vi "Sensor Group 6 to Sensor Group 6 (graphical).vi"(3 "Net Angle (deg)":i32, 4 "Net Dist (mm)":i32, 6 "iRobot Sensor Group 6":T1={"Bumps + Wheel Drops"={"Wheeldrop Caster"=FALSE, "Wheeldrop Left"=FALSE, "Wheeldrop Right"=FALSE, "Bump Left"=FALSE, "Bump Right"=FALSE}, "Wall"=FALSE, "Cliff Left"=FALSE, "Cliff Front Left"=FALSE, "Cliff Front Right"=FALSE, "Cliff Right"=FALSE, "Wall Signal"=0, "Cliff Left Signal"=0, "Cliff Front Left Signal"=0, "Cliff Front Right Signal"=0, "Cliff Right Signal"=0, "Buttons"={"Advance"=FALSE, "Play"=FALSE}, "Virtual Wall"=FALSE, "# Stream Packets"=0, "Requested Velocity (mm/s)"=0, "Requested Radius (mm)"=0, "Requested Right Wheel Velocity (mm/s)"=0, "Requested Left Wheel Velocity (mm/s)"=0, "Distance (mm)"=0, "Angle (deg)"=0, "Song Playing"=FALSE, "Song Number"=0, "Charging State"=enum."Not Charging", "Voltage (mV)"=0, "Current (mA)"=0, "Battery Temperature (deg C)"=0, "Battery Charge (mAh)"=0, "Battery Capacity (mAh)"=0, "Charging Sources"={"Internal Charger"=FALSE, "Home Base"=FALSE}, "OI Mode"=enum."Off", "Digital Inputs"={"Digital Input 0"=FALSE, "Digital Input 1"=FALSE, "Digital Input 2"=FALSE, "Digital Input 3"=FALSE, "Device Detect"=FALSE}, "Drivers & Wheel Overcurrent"={"Low-Side Driver 0"=FALSE, "Low-Side Driver 1"=FALSE, "Low-Side Driver 2"=FALSE, "Left Wheel"=FALSE, "Right Wheel"=FALSE}, "Analog Signal"=0, "Infrared"=255} {"Infrared" format="%02x"}) -> (1 "iRobot Sensors (graphical)":T9={"Caster Wheel Drop"=FALSE, "Left Wheel Drop"=FALSE, "Right Wheel Drop"=FALSE, "Left Bump"=FALSE, "Right Bump"=FALSE, "Left Cliff"=FALSE, "Front Left Cliff"=FALSE, "Front Right Cliff"=FALSE, "Right Cliff"=FALSE, "Wall"=FALSE, "Left Wheel Overcurrent"=FALSE, "Right Wheel Overcurrent"=FALSE, "Infrared"=255, "Play"=FALSE, "Advance"=FALSE, "Net Dist (mm)"=0, "Net Angle (deg)"=0, "Charging State"=enum."Not Charging", "Voltage (mV)"=0, "Current (mA)"=0, "Battery Temperature (C)"=0, "Battery Charge (mAh)"=0, "Battery Capacity (mAh)"=255, "Wall (mm)"=0, "Left Cliff"=0, "Front Left Cliff"=0, "Front Right Cliff"=0, "Right Cliff"=0, "OI Mode"=enum."Off", "Song Number"=0, "Song Playing"=FALSE, "Power"=FALSE, "Left Wheel (mm/s)"=0, "Right Wheel (mm/s)"=0} {"Infrared" format="%02x"; "Right Wheel (mm/s)" scale=-500.0..500.0; "Left Wheel (mm/s)" scale=-500.0..500.0})   [LabVIEW 2014]
uses:
  Sensor Group 6 (graphical).ctl
  Charging State.ctl
  OI Mode.ctl
  Sensor Group 6.ctl
  Bumps + Wheel Drops.ctl
  Buttons.ctl
  Charging Sources Available.ctl
  Cargo Bay Digital Inputs.ctl
  Low-Side Driver + Wheel Overcurrent.ctl
panel:
  # "Electrical: charging, battery, OI mode"
  # "Sensors: bump, cliff, button, wheel drop, wall, virtual wall"
  # "Motion: distance, angle, requested velocity"
  # "Cargo Bay: I/O, overcurrent, infrared"
  # "Song"
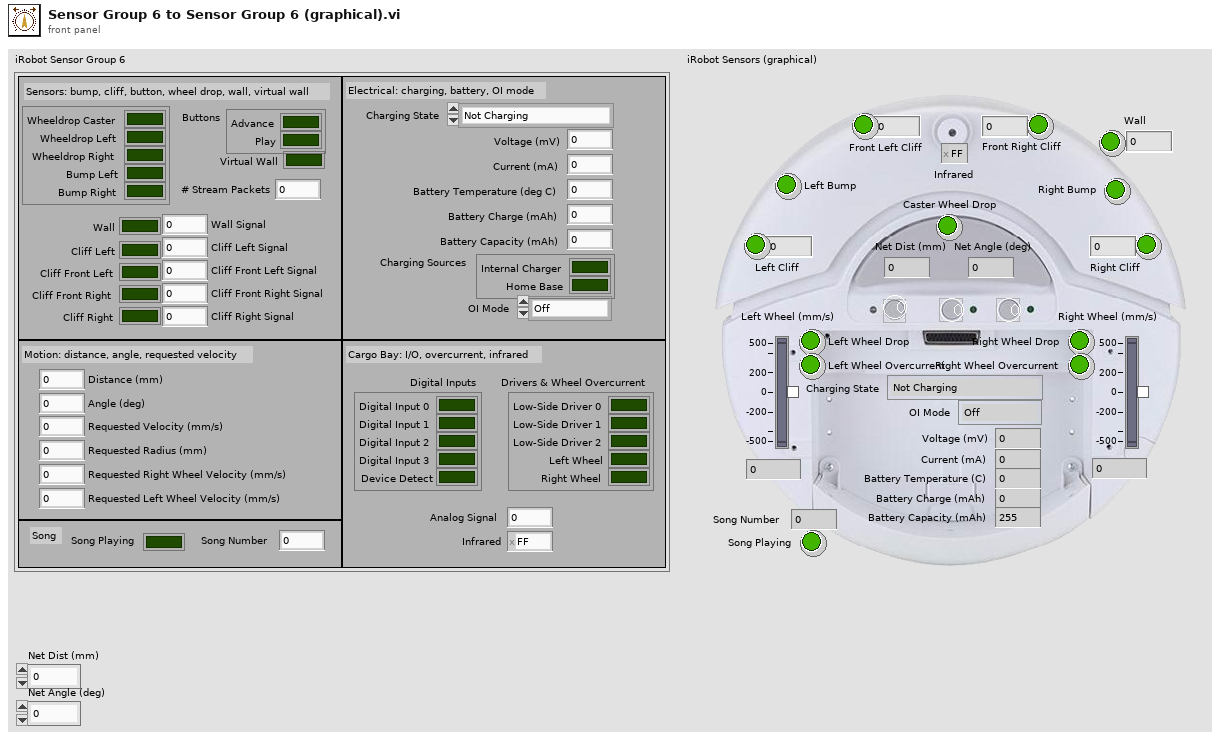
[diagram p1: front panel]
types:
  T1 = typedef "Sensor Group 6.ctl" = cluster{"Bumps + Wheel Drops":T2, "Wall":bool, "Cliff Left":bool, "Cliff Front Left":bool, "Cliff Front Right":bool, "Cliff Right":bool, "Wall Signal":u16, "Cliff Left Signal":u16, "Cliff Front Left Signal":u16, "Cliff Front Right Signal":u16, "Cliff Right Signal":u16, "Buttons":T3, "Virtual Wall":bool, "# Stream Packets":u8, "Requested Velocity (mm/s)":i16, "Requested Radius (mm)":i16, "Requested Right Wheel Velocity (mm/s)":i16, "Requested Left Wheel Velocity (mm/s)":i16, "Distance (mm)":i32, "Angle (deg)":i32, "Song Playing":bool, "Song Number":u8, "Charging State":T4, "Voltage (mV)":u16, "Current (mA)":i16, "Battery Temperature (deg C)":i8, "Battery Charge (mAh)":u16, "Battery Capacity (mAh)":u16, "Charging Sources":T5, "OI Mode":T6, "Digital Inputs":T7, "Drivers & Wheel Overcurrent":T8, "Analog Signal":u16, "Infrared":u8}
  T2 = typedef "Bumps + Wheel Drops.ctl" = cluster{"Wheeldrop Caster":bool, "Wheeldrop Left":bool, "Wheeldrop Right":bool, "Bump Left":bool, "Bump Right":bool}
  T3 = typedef "Buttons.ctl" = cluster{"Advance":bool, "Play":bool}
  T4 = typedef "Charging State.ctl" = enum16{"Not Charging", "Reconditioning Charging", "Full Charging", "Trickle Charging", "Waiting", "Charging Fault Condition"}
  T5 = typedef "Charging Sources Available.ctl" = cluster{"Internal Charger":bool, "Home Base":bool}
  T6 = typedef "OI Mode.ctl" = enum16{"Off", "Passive", "Safe", "Full"}
  T7 = typedef "Cargo Bay Digital Inputs.ctl" = cluster{"Digital Input 0":bool, "Digital Input 1":bool, "Digital Input 2":bool, "Digital Input 3":bool, "Device Detect":bool}
  T8 = typedef "Low-Side Driver + Wheel Overcurrent.ctl" = cluster{"Low-Side Driver 0":bool, "Low-Side Driver 1":bool, "Low-Side Driver 2":bool, "Left Wheel":bool, "Right Wheel":bool}
  T9 = typedef "Sensor Group 6 (graphical).ctl" = cluster{"Caster Wheel Drop":bool, "Left Wheel Drop":bool, "Right Wheel Drop":bool, "Left Bump":bool, "Right Bump":bool, "Left Cliff":bool, "Front Left Cliff":bool, "Front Right Cliff":bool, "Right Cliff":bool, "Wall":bool, "Left Wheel Overcurrent":bool, "Right Wheel Overcurrent":bool, "Infrared":u8, "Play":bool, "Advance":bool, "Net Dist (mm)":i32, "Net Angle (deg)":i32, "Charging State":T4, "Voltage (mV)":u16, "Current (mA)":i16, "Battery Temperature (C)":i8, "Battery Charge (mAh)":u16, "Battery Capacity (mAh)":u16, "Wall (mm)":u16, "Left Cliff":u16, "Front Left Cliff":u16, "Front Right Cliff":u16, "Right Cliff":u16, "OI Mode":T6, "Song Number":u8, "Song Playing":bool, "Power":bool, "Left Wheel (mm/s)":i16, "Right Wheel (mm/s)":i16}
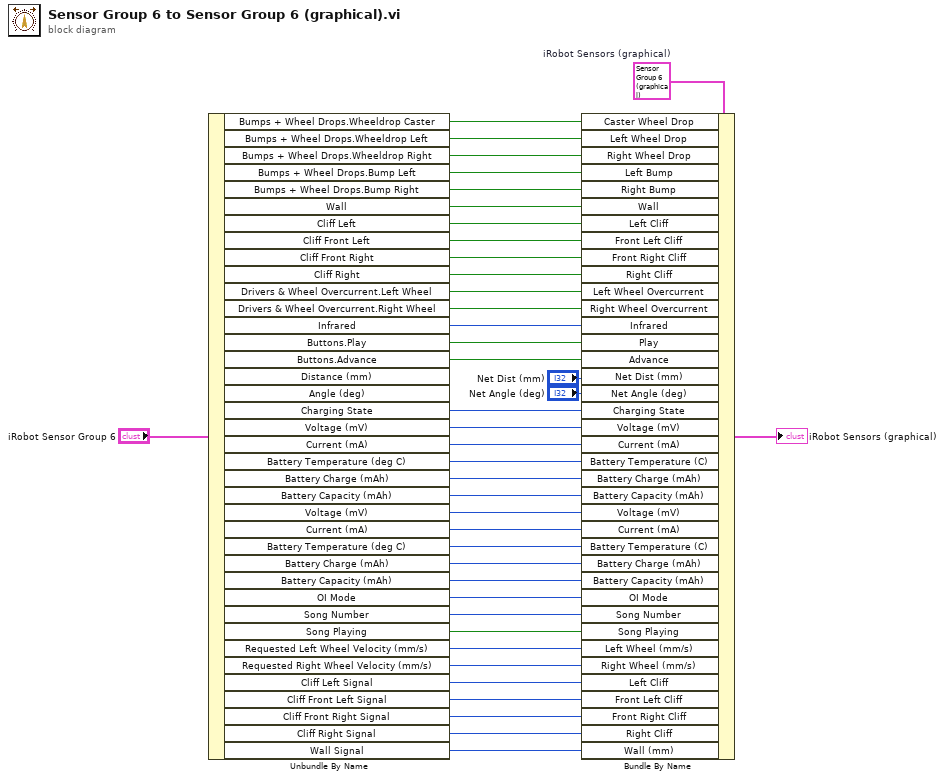
[diagram p0: block diagram]
diagram:
  w40 = T9 {"Caster Wheel Drop"=FALSE, "Left Wheel Drop"=FALSE, "Right Wheel Drop"=FALSE, "Left Bump"=FALSE, "Right Bump"=FALSE, "Left Cliff"=FALSE, "Front Left Cliff"=FALSE, "Front Right Cliff"=FALSE, "Right Cliff"=FALSE, "Wall"=FALSE, "Left Wheel Overcurrent"=FALSE, "Right Wheel Overcurrent"=FALSE, "Infrared"=0, "Play"=FALSE, "Advance"=FALSE, "Net Dist (mm)"=0, "Net Angle (deg)"=0, "Charging State"=enum."Not Charging", "Voltage (mV)"=0, "Current (mA)"=0, "Battery Temperature (C)"=0, "Battery Charge (mAh)"=0, "Battery Capacity (mAh)"=0, "Wall (mm)"=0, "Left Cliff"=0, "Front Left Cliff"=0, "Front Right Cliff"=0, "Right Cliff"=0, "OI Mode"=enum."Off", "Song Number"=0, "Song Playing"=FALSE, "Power"=FALSE, "Left Wheel (mm/s)"=0, "Right Wheel (mm/s)"=0}  # iRobot Sensors (graphical)
  n1 = Unbundle By Name("iRobot Sensor Group 6") -> ("Bumps + Wheel Drops.Wheeldrop Caster"=w39:bool, "Bumps + Wheel Drops.Wheeldrop Left"=w38:bool, "Bumps + Wheel Drops.Wheeldrop Right"=w37:bool, "Bumps + Wheel Drops.Bump Left"=w36:bool, "Bumps + Wheel Drops.Bump Right"=w35:bool, "Wall"=w34:bool, "Cliff Left"=w33:bool, "Cliff Front Left"=w32:bool, "Cliff Front Right"=w31:bool, "Cliff Right"=w30:bool, "Drivers & Wheel Overcurrent.Left Wheel"=w29:bool, "Drivers & Wheel Overcurrent.Right Wheel"=w28:bool, "Infrared"=w27:u8, "Buttons.Play"=w26:bool, "Buttons.Advance"=w25:bool, "Charging State"=w24:T4, "Voltage (mV)"=w23:u16, "Current (mA)"=w22:i16, "Battery Temperature (deg C)"=w21:i8, "Battery Charge (mAh)"=w20:u16, "Battery Capacity (mAh)"=w19:u16, "Voltage (mV)"=w18:u16, "Current (mA)"=w17:i16, "Battery Temperature (deg C)"=w16:i8, "Battery Charge (mAh)"=w15:u16, "Battery Capacity (mAh)"=w14:u16, "OI Mode"=w13:T6, "Song Number"=w12:u8, "Song Playing"=w11:bool, "Requested Left Wheel Velocity (mm/s)"=w10:i16, "Requested Right Wheel Velocity (mm/s)"=w9:i16, "Cliff Left Signal"=w5:u16, "Cliff Front Left Signal"=w4:u16, "Cliff Front Right Signal"=w3:u16, "Cliff Right Signal"=w2:u16, "Wall Signal"=w1:u16)  [unwired: 2 out]
  n2 = Bundle By Name(cluster=w40, "Caster Wheel Drop"=w39, "Left Wheel Drop"=w38, "Right Wheel Drop"=w37, "Left Bump"=w36, "Right Bump"=w35, "Wall"=w34, "Left Cliff"=w33, "Front Left Cliff"=w32, "Front Right Cliff"=w31, "Right Cliff"=w30, "Left Wheel Overcurrent"=w29, "Right Wheel Overcurrent"=w28, "Infrared"=w27, "Play"=w26, "Advance"=w25, "Net Dist (mm)"="Net Dist (mm)", "Net Angle (deg)"="Net Angle (deg)", "Charging State"=w24, "Voltage (mV)"=w23, "Current (mA)"=w22, "Battery Temperature (C)"=w21, "Battery Charge (mAh)"=w20, "Battery Capacity (mAh)"=w19, "Voltage (mV)"=w18, "Current (mA)"=w17, "Battery Temperature (C)"=w16, "Battery Charge (mAh)"=w15, "Battery Capacity (mAh)"=w14, "OI Mode"=w13, "Song Number"=w12, "Song Playing"=w11, "Left Wheel (mm/s)"=w10, "Right Wheel (mm/s)"=w9, "Left Cliff"=w5, "Front Left Cliff"=w4, "Front Right Cliff"=w3, "Right Cliff"=w2, "Wall (mm)"=w1) -> (→"iRobot Sensors (graphical)":T9)
